vi "GFITS_dhs_server.vi"(9 "cmdport 2":u16, 10 "cmdport":u16) -> ()   [LabVIEW 2016]
doc: "Main VI for the COMSTCP Module. This module is in charge of the externl TCP/IP comunications"
uses:
  DRV_DHS/private/vis/DRV_DHS_CmdStruct.ctl
  DHS_TCPSERVER_MsgStruct.ctl
panel:
  out "singport 2":u16=1502
  in  "ResponseStruct":T1
  in  "dhscmdstruct":T2
  out "last response":string
  out "singport":u16=1502
  out "stopped":bool=TRUE
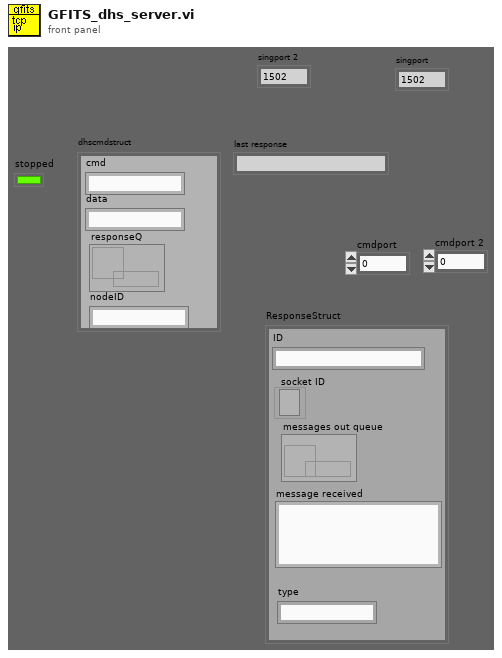
[diagram p1: front panel]
types:
  T1 = typedef "DHS_TCPSERVER_MsgStruct.ctl" = cluster{"ID":string, "socket ID":refnum<k5>, "messages out queue":refnum<queue>, "message received":string, "type":string}
  T2 = typedef "DRV_DHS_CmdStruct.ctl" = cluster{"cmd":string, "data":string, "responseQ":refnum<queue>, "nodeID":string}
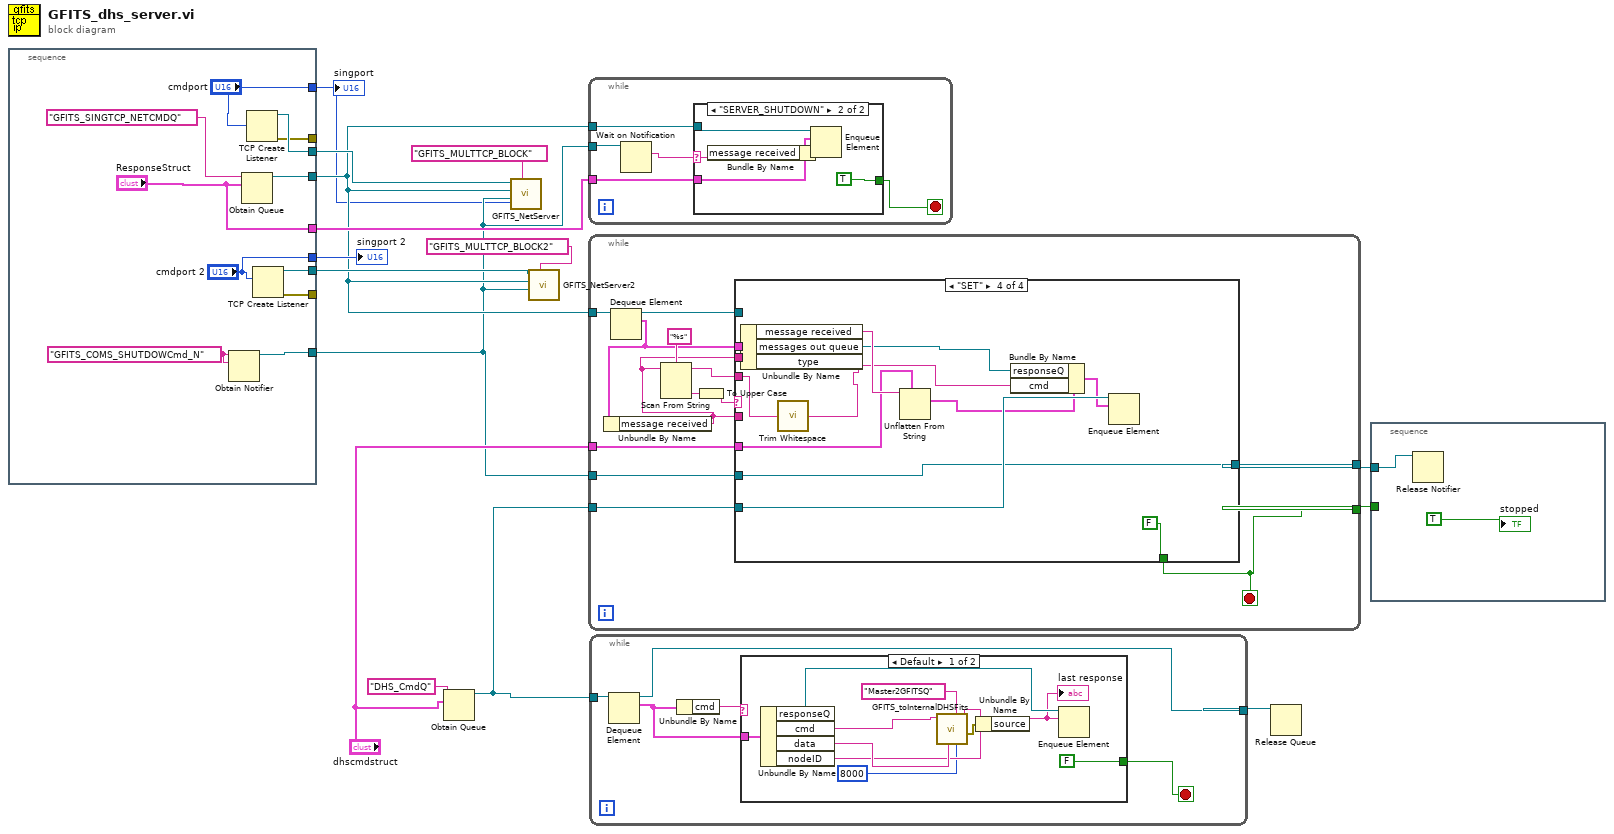
[diagram p0: block diagram]
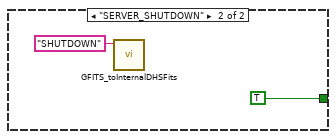
[diagram p2: hidden frame]
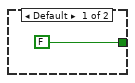
[diagram p3: hidden frame]
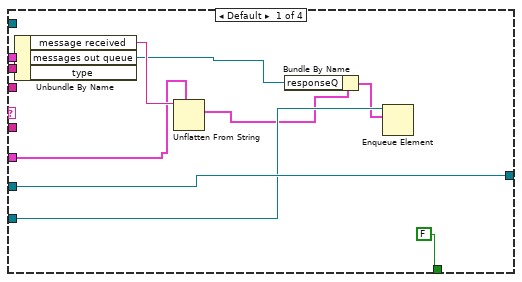
[diagram p4: hidden frame]
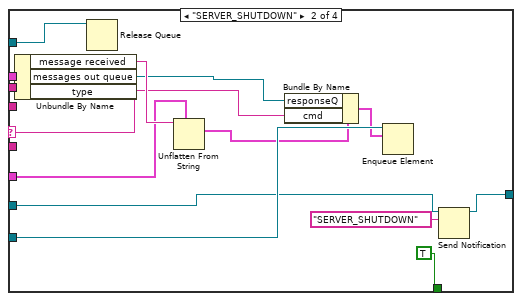
[diagram p5: hidden frame]
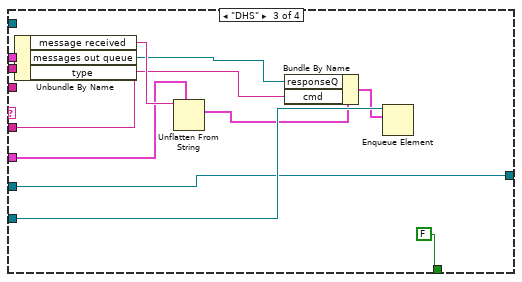
[diagram p6: hidden frame]
diagram:
  n1 = stacked-sequence {
    tunnel: [w25] -> w2
    tunnel: ["cmdport"] -> w1
    tunnel: [w23] -> w13
    tunnel: [w22] -> w3
    tunnel: ["ResponseStruct"] -> w11
    tunnel: [w19] -> w5
    tunnel: ["cmdport 2"] -> w6
    tunnel: [w17] -> _
    tunnel: [w16] -> _
    frame #0 {
      w26 = "GFITS_COMS_SHUTDOWCmd_N" ("name (unnamed)")
      n2 = Obtain Notifier(name (unnamed)=w26, notification data type=w26) -> (notifier out=w25:refnum<notifier>)  [unwired: 2 in, 2 out]
      n3 = Obtain Queue(name (unnamed)="GFITS_SINGTCP_NETCMDQ" ("messages from socks Q name"), element data type="ResponseStruct") -> (queue out=w22:refnum<queue>)  [unwired: 3 in, 2 out]
      n4 = TCP Create Listener(10:"cmdport") -> (0:w17:errorcluster, 3:w23:refnum<k5>)  [unwired: 1 in, 4 out]
      n5 = TCP Create Listener(10:"cmdport 2") -> (0:w16:errorcluster, 3:w19:refnum<k5>)  [unwired: 1 in, 4 out]
    }
  }
  "singport" <- w1
  "singport 2" <- w6
  n6 = Obtain Queue(name (unnamed)="DHS_CmdQ", element data type="dhscmdstruct") -> (queue out=w8:refnum<queue>)  [unwired: 3 in, 2 out]
  n7 = call "GFITS_NetServer.vi"("port"=w1, "ID"="GFITS_MULTTCP_BLOCK", "notifier In"=w2, "messages from sock"=w3, "listener ID"=w13) -> ()  [unwired: 1 in, 6 out]
  n8 = call "GFITS_NetServer2.vi"("ID"="GFITS_MULTTCP_BLOCK2", "notifier In"=w2, "messages from sock"=w3, "listener ID"=w5) -> ()  [unwired: 1 in, 7 out]
  n9 = while {
    tunnel: w2 -> [w31]
    tunnel: w3 -> [w28]
    tunnel: w11 -> [w27]
    stop <- w29 stop-if-true
    n10 = Wait on Notification(notifier=w31) -> (notification=w30:string)  [unwired: 1 in, 5 out]
    n11 = case shown="\"SERVER_SHUTDOWN\"" w30 {
      selector: w30 -> [_ w33]
      tunnel: [FALSE TRUE] -> w29
      tunnel: w28 -> [_ w36]
      tunnel: w27 -> [_ w35]
      frame Default {
      }
      frame "SERVER_SHUTDOWN" {
        n12 = Bundle By Name(cluster=w35, "message received"=w33) -> (w34:T1)
        n13 = Enqueue Element(queue=w36, element=w34) -> ()  [unwired: 1 in, 4 out]
      }
    }
  }
  n14 = while {
    tunnel: [w44] -> w15
    tunnel: w2 -> [w43]
    tunnel: [w42] -> w14
    tunnel: w3 -> [w41]
    tunnel: w8 -> [w40]
    tunnel: "dhscmdstruct" -> [w39]
    stop <- w44 stop-if-true
    n15 = Dequeue Element(queue=w41) -> (queue out=w46:refnum<queue>, element=w45:T1)  [unwired: 1 in, 3 out]
    n16 = Unbundle By Name(w45) -> ("message received"=w38:string)
    n17 = Scan From String(format string="%s", input string=w38) -> (remaining string=w48:string, output 1=w47:string)  [unwired: 2 in, 3 out]
    n18 = To Upper Case(1:w47) -> (0:w49:string)
    n19 = case shown="\"SET\"" w49 {
      selector: w49 -> [_ w60 _ _]
      tunnel: [FALSE TRUE FALSE FALSE] -> w44
      tunnel: w45 -> [w59 w72 w82 w93]
      tunnel: w48 -> [_ _ _ w84]
      tunnel: w46 -> [_ w65 _ _]
      tunnel: w38 -> [_ _ _ _]
      tunnel: w43 -> [w57 w63 w74 w85]
      tunnel: [w57 w62 w74 w85] -> w42
      tunnel: w40 -> [w55 w69 w79 w90]
      tunnel: w39 -> [w51 w61 w75 w86]
      tunnel: w38 -> [_ _ w73 _]
      frame Default {
        n20 = Unbundle By Name(w59) -> ("message received"=w56:string, "messages out queue"=w53:refnum<queue>)  [unwired: 1 out]
        n21 = Unflatten From String(type=w51, binary string=w56) -> (value=w54:T2)  [unwired: 1 in, 4 out]
        n22 = Bundle By Name(cluster=w54, "responseQ"=w53) -> (w52:T2)
        n23 = Enqueue Element(queue=w55, element=w52) -> ()  [unwired: 1 in, 4 out]
      }
      frame "SERVER_SHUTDOWN" {
        n24 = Unbundle By Name(w72) -> ("message received"=w70:string, "messages out queue"=w67:refnum<queue>)  [unwired: 1 out]
        n25 = Release Queue(queue=w65) -> ()  [unwired: 1 in, 4 out]
        n26 = Unflatten From String(type=w61, binary string=w70) -> (value=w68:T2)  [unwired: 1 in, 4 out]
        n27 = Bundle By Name(cluster=w68, "responseQ"=w67, "cmd"=w60) -> (w66:T2)
        n28 = Enqueue Element(queue=w69, element=w66) -> ()  [unwired: 1 in, 4 out]
        n29 = Send Notification(notification="SERVER_SHUTDOWN", notifier=w63) -> (notifier out=w62:refnum<notifier>)  [unwired: 1 in, 1 out]
      }
      frame "DHS" {
        n30 = Unbundle By Name(w82) -> ("message received"=w80:string, "messages out queue"=w77:refnum<queue>)  [unwired: 1 out]
        n31 = Unflatten From String(type=w75, binary string=w80) -> (value=w78:T2)  [unwired: 1 in, 4 out]
        n32 = Bundle By Name(cluster=w78, "responseQ"=w77, "cmd"=w73) -> (w76:T2)
        n33 = Enqueue Element(queue=w79, element=w76) -> ()  [unwired: 1 in, 4 out]
      }
      frame "SET" {
        n34 = Unbundle By Name(w93) -> ("message received"=w91:string, "messages out queue"=w88:refnum<queue>)  [unwired: 1 out]
        n35 = call <vilib>:"Trim Whitespace.vi"("string"=w84) -> ("trimmed string"=w83:string)  [unwired: 1 in]
        n36 = Unflatten From String(type=w86, binary string=w91) -> (value=w89:T2)  [unwired: 1 in, 4 out]
        n37 = Bundle By Name(cluster=w89, "responseQ"=w88, "cmd"=w83) -> (w87:T2)
        n38 = Enqueue Element(queue=w90, element=w87) -> ()  [unwired: 1 in, 4 out]
      }
    }
  }
  n39 = while {
    tunnel: w8 -> [w98]
    tunnel: [w95] -> w9
    stop <- w96 stop-if-true
    n40 = Dequeue Element(queue=w98) -> (queue out=w95:refnum<queue>, element=w94:T2)  [unwired: 1 in, 3 out]
    n41 = Unbundle By Name(w94) -> ("cmd"=w97:string)
    n42 = case shown="Default" w97 {
      tunnel: [FALSE TRUE] -> w96
      tunnel: w94 -> [w104 _]
      frame Default {
        n43 = Unbundle By Name(w104) -> ("responseQ"=w101:refnum<queue>, "cmd"=w99:string, "data"=w107:string, "nodeID"=w103:string)
        n44 = call "GFITS_toInternalDHSFits.vi"("nodeID"=w103, "ms timeout (-1)"=8000, "response Q"="Master2GFITSQ", "key"=w107, "command"=w99) -> ("response"=w108:errorcluster)  [unwired: 1 in, 5 out]
        n45 = Unbundle By Name(w108) -> ("source"=w100:string)
        "last response" <- w100
        n46 = Enqueue Element(queue=w101, element=w100) -> ()  [unwired: 2 in, 3 out]
      }
      frame "SERVER_SHUTDOWN" {
        n47 = call "GFITS_toInternalDHSFits.vi"("command"="SHUTDOWN") -> ()  [unwired: 5 in, 6 out]
      }
    }
  }
  n48 = Release Queue(queue=w9) -> ()  [unwired: 1 in, 4 out]
  n49 = stacked-sequence {
    tunnel: w15 -> [_]
    tunnel: w14 -> [w111]
    frame #0 {
      n50 = Release Notifier(notifier=w111) -> ()  [unwired: 1 in, 4 out]
      "stopped" <- TRUE
    }
  }
